vi "SetCommandValue.vi"(3 "error in (no error)":errorcluster, 4 "strName":string, 5 "nInputHandle":u64) -> (0 "error out":errorcluster, 1 "GX_STATUS":i32, 2 "nOutputHandle":u64)   [LabVIEW 2016, in "GxLVLib.lvlib"]
uses:
  GxLVLib.lvlib
  GxIAPI.dll
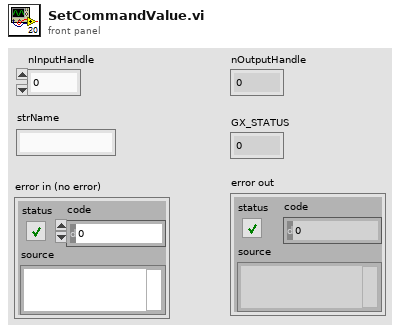
[diagram p1: front panel]
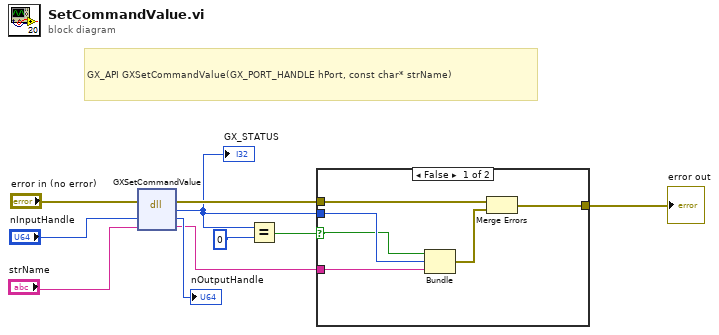
[diagram p0: block diagram]
diagram:
  # "GX_API GXSetCommandValue(GX_PORT_HANDLE hPort, const char* strName)"
  n1 = dll-call lib="GxIAPI.dll" fn="GXSetCommandValue"(error in="error in (no error)", "hDevice"="nInputHandle", "strName"="strName") -> (error out=w5:errorcluster, "GX_STATUS"=w2:i32, "hDevice"=→"nOutputHandle":i64, "strName"=w1:string)  [unwired: 2 in, 1 out]
  "GX_STATUS" <- w2
  n2 = Equal?(x=w2, y=0) -> (x = y?=w4:bool)
  n3 = case shown="False" w4 {
    selector: w4 -> [w11 _]
    tunnel: w5 -> [w16 w17]
    tunnel: [w15 w17] -> w6
    tunnel: w2 -> [w13 _]
    tunnel: w1 -> [w12 _]
    frame False {
      n4 = Bundle(w11, "GX_STATUS"=w13, "strName"=w12) -> (w14:cluster{bool, "GX_STATUS":i32, "strName":string})  [unwired: 1 in]
      n5 = Merge Errors(w16, w14) -> (w15:errorcluster)
    }
    frame True {
    }
  }
  "error out" <- w6
